vi "Caveat 2 Fix.vi"() -> ()   [LabVIEW 2025]
panel:
  out "Loop Iterations":i32
  out "Startup Msg":string
  # "Caveat #2: UI Only Updates when Remote Panel Connection Active (Must Explicitly Refresh by Writing to Each Indicator)"
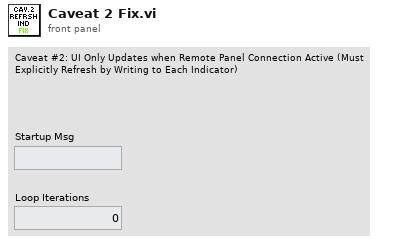
[diagram p1: front panel]
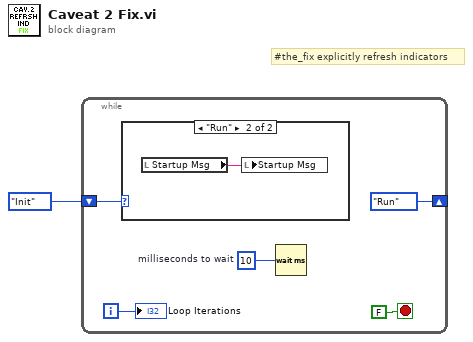
[diagram p0: block diagram]
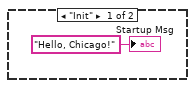
[diagram p2: hidden frame]
diagram:
  # "#the_fix explicitly refresh indicators"
  n1 = while {
    shift-right: [enum16{"Init", "Run"}."Run"] -> _
    shift-left: enum16{"Init", "Run"}."Init" -> [w4]
    i -> [w2]
    stop <- FALSE stop-if-true
    w5 = u32 10  # milliseconds to wait
    n2 = case shown="\"Run\"" w4 {
      frame "Init" {
        "Startup Msg" <- "Hello, Chicago!" ("Msg Written Only at Startup")
      }
      frame "Run" {
        n3 = local read "Startup Msg"() -> (w8:string)
        n4 = local write "Startup Msg"(w8) -> ()
      }
    }
    n5 = Wait (ms)(milliseconds to wait=w5) -> ()  [unwired: 1 out]
    "Loop Iterations" <- w2
  }
